vi "Lab1.vi"() -> ()   [LabVIEW 2011]
panel:
  out "z2":dbl
  out "z1":dbl
  out "y2":dbl
  out "y1":dbl
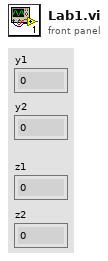
[diagram p1: front panel]
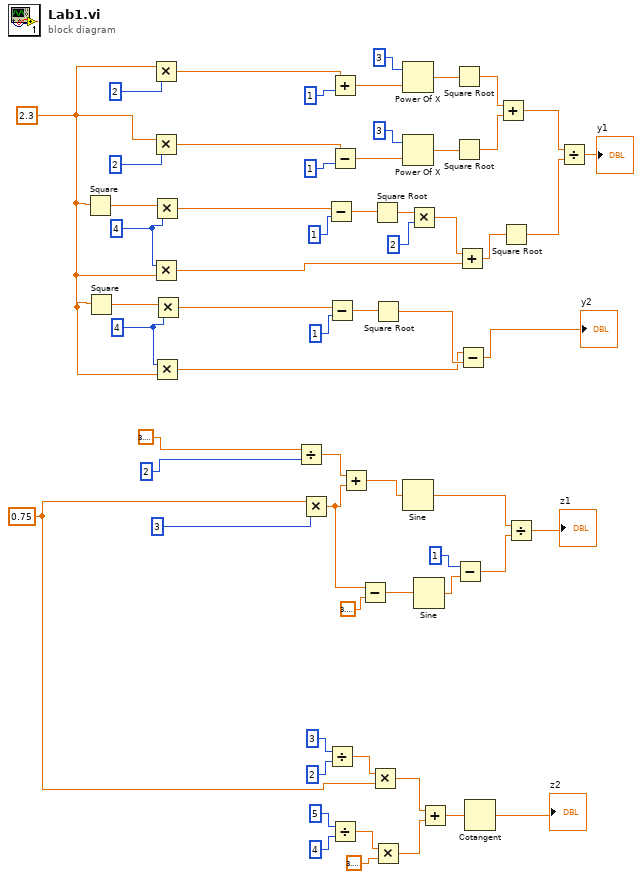
[diagram p0: block diagram]
diagram:
  w30 = 4
  w41 = 4
  w29 = 2.3
  w9 = 0.75
  n1 = Square(x=w29) -> (x^2=w44:dbl)
  n2 = Square(x=w29) -> (x^2=w31:dbl)
  n3 = Multiply(x=w29, y=2) -> (x*y=w60:dbl)
  n4 = Multiply(x=w29, y=2) -> (x*y=w54:dbl)
  n5 = Multiply(x=w41, y=w29) -> (x*y=w40:dbl)
  n6 = Multiply(x=w44, y=w41) -> (x*y=w47:dbl)
  n7 = Multiply(x=w30, y=w29) -> (x*y=w27:dbl)
  n8 = Multiply(x=w31, y=w30) -> (x*y=w34:dbl)
  n9 = Divide(x=3.141592653589793, y=2) -> (x/y=w22:dbl)
  n10 = Multiply(x=w9, y=3) -> (x*y=w18:dbl)
  n11 = Subtract(x=w47, y=1) -> (x-y=w45:dbl)
  n12 = Subtract(x=w34, y=1) -> (x-y=w32:dbl)
  n13 = Divide(x=3, y=2) -> (x/y=w10:dbl)
  n14 = Add(x=w60, y=1) -> (x+y=w58:dbl)
  n15 = Subtract(x=w54, y=1) -> (x-y=w52:dbl)
  n16 = Divide(x=5, y=4) -> (x/y=w6:dbl)
  n17 = Add(x=w22, y=w18) -> (x+y=w21:dbl)
  n18 = Subtract(x=w18, y=3.141592653589793) -> (x-y=w16:dbl)
  n19 = Multiply(x=w10, y=w9) -> (x*y=w3:dbl)
  n20 = Square Root(x=w45) -> (sqrt(x)=w43:dbl)
  n21 = Square Root(x=w32) -> (sqrt(x)=w28:dbl)
  n22 = Multiply(x=w6, y=3.141592653589793) -> (x*y=w2:dbl)
  n23 = Power Of X(1:w58, 2:3) -> (0:w56:dbl)
  n24 = Power Of X(1:w52, 2:3) -> (0:w50:dbl)
  n25 = Sine(x=w21) -> (sin(x)=w15:dbl)
  n26 = Multiply(x=w43, y=2) -> (x*y=w39:dbl)
  n27 = Sine(x=w16) -> (sin(x)=w20:dbl)
  n28 = Add(x=w3, y=w2) -> (x+y=w4:dbl)
  n29 = Square Root(x=w56) -> (sqrt(x)=w49:dbl)
  n30 = Square Root(x=w50) -> (sqrt(x)=w48:dbl)
  n31 = Subtract(x=1, y=w20) -> (x-y=w14:dbl)
  n32 = Add(x=w39, y=w40) -> (x+y=w38:dbl)
  n33 = Subtract(x=w27, y=w28) -> (x-y=→"y2":dbl)
  n34 = Cotangent(1:w4) -> (0:→"z2":dbl)
  n35 = Add(x=w49, y=w48) -> (x+y=w37:dbl)
  n36 = Square Root(x=w38) -> (sqrt(x)=w36:dbl)
  n37 = Divide(x=w15, y=w14) -> (x/y=→"z1":dbl)
  n38 = Divide(x=w37, y=w36) -> (x/y=→"y1":dbl)
